vi "20220114_04_Test.vi"() -> ()   [LabVIEW 2019]
uses:
  20220114_04_Function.ctl
panel:
  in  "Run":bool
  out "Output":dbl
  in  "Function":T1
  in  "Stop":bool
  in  "Input":dbl
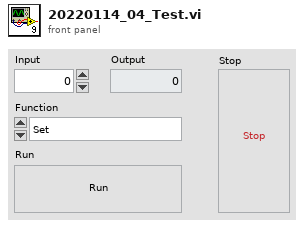
[diagram p1: front panel]
types:
  T1 = typedef "20220114_04_Function.ctl" = enum16{"Set", "Get", "Reset"}
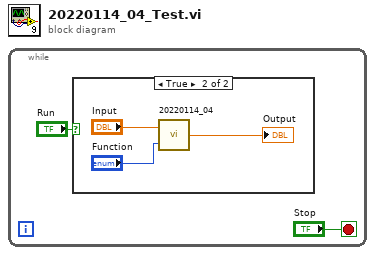
[diagram p0: block diagram]
diagram:
  n1 = while {
    stop <- "Stop" stop-if-true
    n2 = case shown="True" "Run" {
      frame False {
      }
      frame True {
        n3 = call "20220114_04.vi"("Function"="Function", "Input"="Input") -> ("Output"=→"Output":dbl)
      }
    }
  }
